vi "Emergency Send To Specific Target.vi"(8 "error in (no error)":errorcluster, 9 "Mail Strategy In":refnum<class "Mail Strategy.lvclass">, 10 "Message In":refnum<class "Message.lvclass">, 11 "Messenger in":refnum<class "Simple Tree Queue Messenger.lvclass">) -> (0 "error out":errorcluster, 3 "Messenger out":refnum<class "Simple Tree Queue Messenger.lvclass">)   [LabVIEW 2019, in "Simple Tree Queue Messenger.lvclass"]
uses:
  Simple Tree Queue Messenger.lvclass
  C:/Users/iio/Desktop/NTHU Brain Center/General Library/Ancestor Class/Messenger/Messenger Composite/Messenger Composite.lvclass
  Ancestor Class/Message/Message.lvclass
  Ancestor Class/Messenger/Mail Strategy/Mail Strategy.lvclass
  Simple Tree Queue Mailman/Simple Tree Queue Mailman.lvclass
  C:/Users/iio/Desktop/NTHU Brain Center/General Library/Ancestor Class/Messenger/Mail Strategy/Mail Strategy.lvclass
  Ancestor Class/Messenger/Messenger Composite/Messenger Composite.lvclass/Messenger Composite.ctl
  Simple Tree Queue Mailman/Simple Tree Queue Mailman.lvclass/Simple Tree Queue Mailman.ctl
  Simple Tree Queue Messenger.lvclass/Simple Tree Queue Messenger.ctl
  Simple Tree Queue Mailman/Public Data/Write Address Recursive Access.vi
  Ancestor Class/Messenger/Messenger Composite/Public Data/Read Nodes.vi
  Ancestor Class/Messenger/Messenger/Messenger.lvclass
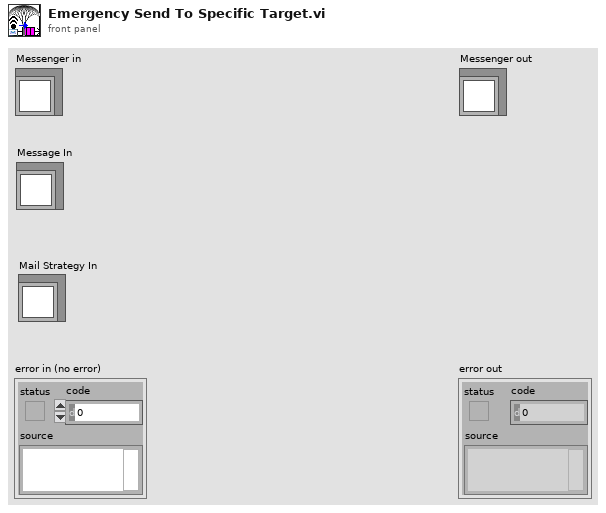
[diagram p1: front panel]
types:
  T1 = typedef "Message Queue.ctl" = refnum<queue>
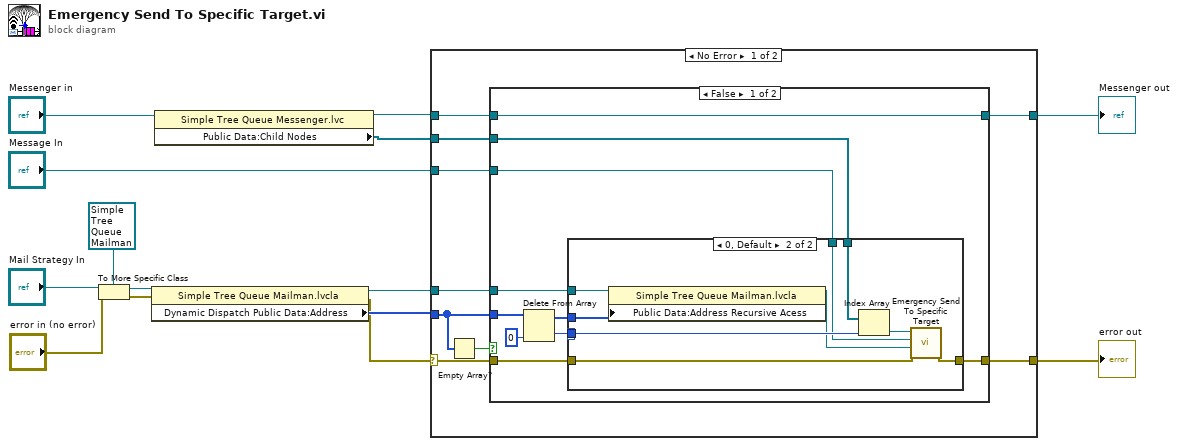
[diagram p0: block diagram]
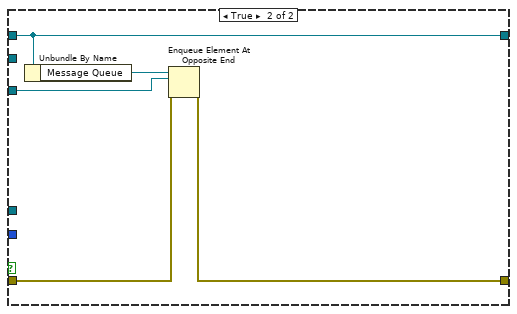
[diagram p3: hidden frame]
diagram:
  n1 = To More Specific Class(target class=refnum<class "Simple Tree Queue Mailman.lvclass"> refnum ("Array Location Mailman.lvclass"), reference="Mail Strategy In", error in="error in (no error)") -> (specific class reference=w7:refnum<class "Simple Tree Queue Mailman.lvclass">, error out=w8:errorcluster)
  n2 = property class="Simple Tree Queue Mailman.lvcla"(reference=w7, error in=w8) -> (reference out=w4:refnum<class "Simple Tree Queue Mailman.lvclass">, error out=w5:errorcluster, "Dynamic Dispatch Public Data:Address"=w6:i32[])
  n3 = property class="Simple Tree Queue Messenger.lvc"(reference="Messenger in") -> (reference out=w2:refnum<class "Simple Tree Queue Messenger.lvclass">, "Public Data:Child Nodes"=w1:refnum<class "Messenger.lvclass">[])  [unwired: 1 in, 1 out]
  n4 = case shown="No Error" w5 {
    selector: w5 -> [w18 w49]
    tunnel: w2 -> [w22 w50]
    tunnel: [w20 w50] -> w14
    tunnel: [w17 w49] -> w12
    tunnel: w6 -> [w19 _]
    tunnel: "Message In" -> [w21 _]
    tunnel: w4 -> [w15 _]
    tunnel: w1 -> [w16 _]
    frame No Error {
      n5 = Empty Array?(array=w19) -> (empty?=w23:bool)
      n6 = case shown="False" w23 {
        tunnel: w22 -> [w33 w48]
        tunnel: w21 -> [w30 w46]
        tunnel: [w33 w48] -> w20
        tunnel: w19 -> [w32 _]
        tunnel: w18 -> [w29 w45]
        tunnel: [w28 w44] -> w17
        tunnel: w16 -> [w27 _]
        tunnel: w15 -> [w25 _]
        frame False {
          n7 = Delete From Array(array=w32, index=0) -> (deleted portion=w24:i32, array with subset deleted=w26:i32[])  [unwired: 1 in]
          n8 = case shown="0, Default" w24 {
            tunnel: w24 -> [_ w43]
            tunnel: w30 -> [_ w41]
            tunnel: w29 -> [w34 w40]
            tunnel: [w34 w39] -> w28
            tunnel: w27 -> [_ w38]
            tunnel: w26 -> [_ w37]
            tunnel: w25 -> [_ w36]
            frame -2147483648..-1 {
            }
            frame 0, Default {
              n9 = property class="Simple Tree Queue Mailman.lvcla"(reference=w36, "Public Data:Address Recursive Acess"=w37) -> (reference out=w35:refnum<class "Simple Tree Queue Mailman.lvclass">)  [unwired: 1 in, 1 out]
              n10 = Index Array(array=w38, index=w43) -> (element=w42:refnum<class "Messenger.lvclass">)
              n11 = call-dynamic "Emergency Send To Specific Target.vi"("error in (no error)"=w40, "Mail Strategy In"=w35, "Message In"=w41, "Messenger in"=w42) -> ("error out"=w39:errorcluster)  [unwired: 6 in, 1 out]
            }
          }
        }
        frame True {
          n12 = Unbundle By Name(w48) -> ("Message Queue"=w47:T1)
          n13 = Enqueue Element At Opposite End(queue=w47, element=w46, error in (no error)=w45) -> (error out=w44:errorcluster)  [unwired: 1 in, 2 out]
        }
      }
    }
    frame Error {
    }
  }
  "error out" <- w12
  "Messenger out" <- w14
